vi "Agilent VNA Read Measurement.vi"(6 "Channel":i8=1 min=1 max=99 step=1, 7 "Agilent VNA":T2, 8 "error in (no error)":errorcluster, 11 "VISA Resource Name":refnum<visa-resource-name>) -> (0 "error out":errorcluster, 1 "Parameter":T1 {"Stimulus Port" min=1 step=1; "Response Port" min=1 step=1}, 2 "Measurement":T3=enum."Analog In - Aux In", 3 "dup VISA Resource Name":refnum<visa-resource-name>)   [LabVIEW 2011]
doc: "This VI for the HP 8753B is used to read the meausurement format.\n\n0 log magnitude\n1 phase\n2 delay\n3 Smith chart\n4 polar\n5 linear magnitude\n6 standing wave ratio\n7 real\n8 imaginary"
uses:
  TypeDefs/Agilent VNA Measurement.ctl
  TypeDefs/Agilent VNA Instrument Info.ctl
  tests/S Parameter/TypeDefs/SP Parameter.ctl
panel:
  in  "Trace":i8=1 min=1 max=99 step=1
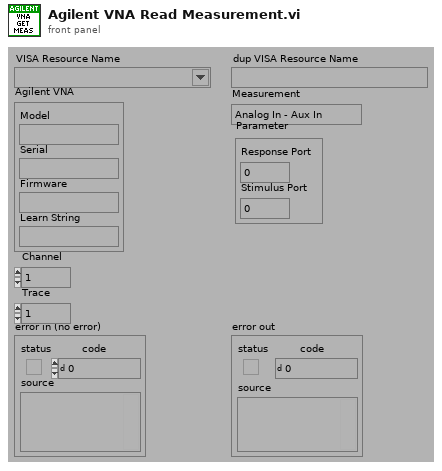
[diagram p1: front panel]
types:
  T1 = typedef "SP Parameter.ctl" = cluster{"Stimulus Port":i8, "Response Port":i8}
  T2 = typedef "Agilent VNA Instrument Info.ctl" = cluster{"Model":string, "Serial":string, "Firmware":string, "Learn String":string}
  T3 = typedef "Agilent VNA Measurement.ctl" = enum32{"SXX", "Analog In - Aux In", "A/R", "B/R", "A/B", "A", "B", "R"}
  T4 = typedef "Agilent VNA Model.ctl" = enum16{"Not Supported", "8510X", "8719X", "8720X", "8722X", "8753X", "ENA", "PNA", "Field Fox"}
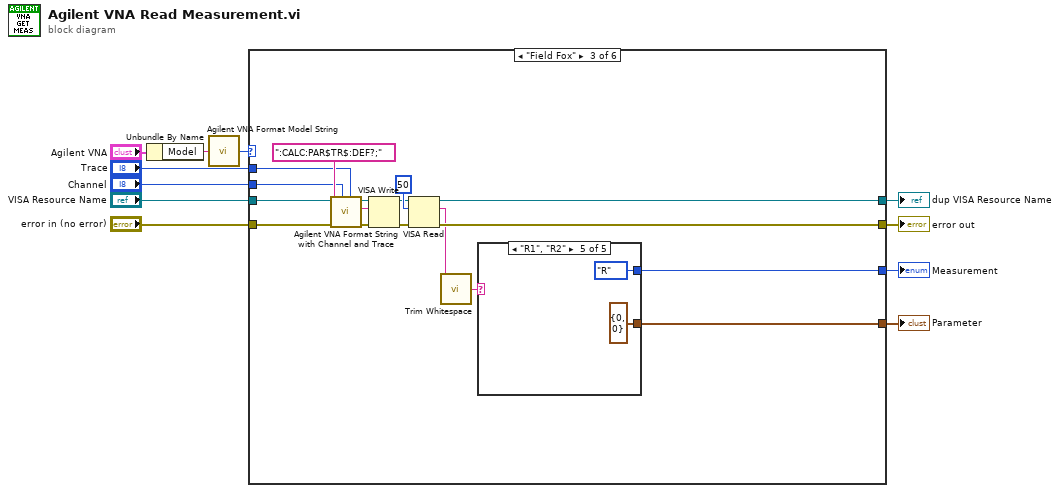
[diagram p0: block diagram]
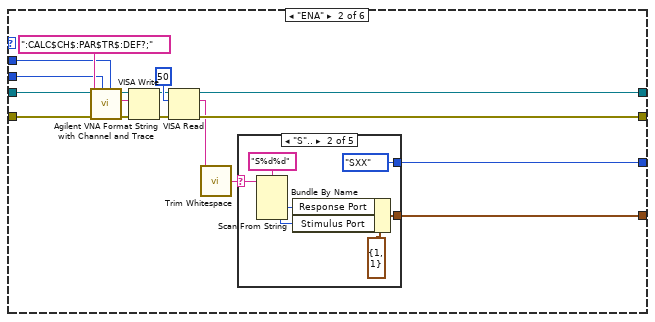
[diagram p3: hidden frame]
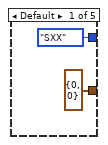
[diagram p4: hidden frame]
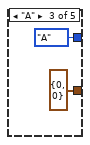
[diagram p5: hidden frame]
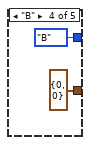
[diagram p6: hidden frame]
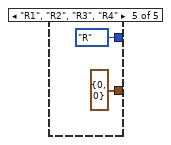
[diagram p7: hidden frame]
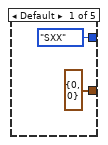
[diagram p8: hidden frame]
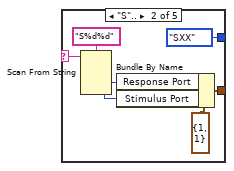
[diagram p9: hidden frame]
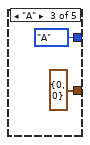
[diagram p10: hidden frame]
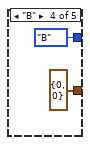
[diagram p11: hidden frame]
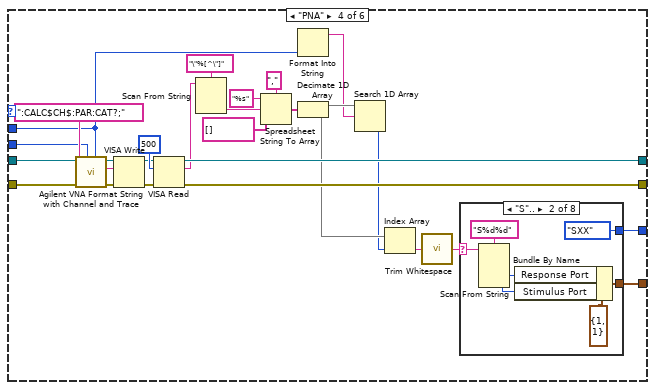
[diagram p12: hidden frame]
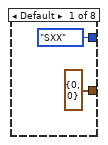
[diagram p13: hidden frame]
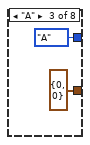
[diagram p14: hidden frame]
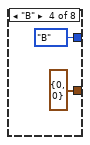
[diagram p15: hidden frame]
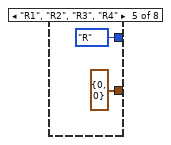
[diagram p16: hidden frame]
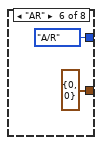
[diagram p17: hidden frame]
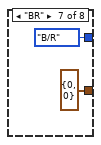
[diagram p18: hidden frame]
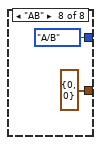
[diagram p19: hidden frame]
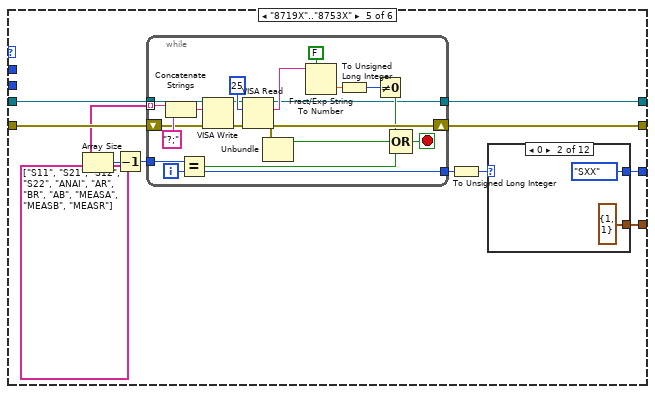
[diagram p20: hidden frame]
diagram:
  n1 = Unbundle By Name("Agilent VNA") -> ("Model"=w2:string)
  n2 = call "Agilent VNA Format Model String.vi"("Model"=w2) -> ("Model"=w6:T4)
  n3 = case shown="\"Field Fox\"" w6 {
    tunnel: "VISA Resource Name" -> [w12 w22 w52 w93 w131 w188]
    tunnel: "error in (no error)" -> [w13 w26 w56 w97 w130 w187]
    tunnel: [w13 w24 w54 w95 w127 w186] -> w9
    tunnel: [_ w17 w47 w75 w122 w177] -> w8
    tunnel: [w12 w23 w53 w94 w124 w185] -> w7
    tunnel: "Channel" -> [_ w16 w46 w78 _ _]
    tunnel: "Trace" -> [_ w15 w45 w77 _ _]
    tunnel: [_ w14 w44 w76 w123 w178] -> w1
    frame "Not Supported" {
    }
    frame "ENA" {
      n4 = call "Agilent VNA Format String with Channel and Trace.vi"("Trace"=w15, "Channel"=w16, "String"=":CALC$CH$:PAR$TR$:DEF?;") -> ("String Out"=w20:string)  [unwired: 6 out]
      n5 = VISA Write(VISA resource name=w22, write buffer=w20, error in (no error)=w26) -> (VISA resource name out=w27:refnum<visa-resource-name>, error out=w25:errorcluster)  [unwired: 1 out]
      n6 = VISA Read(VISA resource name=w27, byte count=u32 50, error in (no error)=w25) -> (VISA resource name out=w23:refnum<visa-resource-name>, read buffer=w19:string, error out=w24:errorcluster)  [unwired: 1 out]
      n7 = call <vilib>:"Trim Whitespace.vi"("string"=w19) -> ("trimmed string"=w18:string)  [unwired: 1 in]
      n8 = case shown="\"S\".." w18 {
        selector: w18 -> [_ w36 _ _ _]
        tunnel: [Agilent_VNA_Measurement."SXX" ("Display Format") Agilent_VNA_Measurement."SXX" ("Display Format") Agilent_VNA_Measurement."A" ("Display Format") Agilent_VNA_Measurement."B" ("Display Format") Agilent_VNA_Measurement."R" ("Display Format")] -> w17
        tunnel: [T1 {"Stimulus Port"=0, "Response Port"=0} ("Parameter") w33 T1 {"Stimulus Port"=0, "Response Port"=0} ("Parameter") T1 {"Stimulus Port"=0, "Response Port"=0} ("Parameter") T1 {"Stimulus Port"=0, "Response Port"=0} ("Parameter")] -> w14
        frame Default {
        }
        frame "S".. {
          n9 = Scan From String(format string="S%d%d", input string=w36) -> (output 1=w32:i32, output 2=w31:i32)  [unwired: 2 in, 5 out]
          n10 = Bundle By Name(cluster=T1 {"Stimulus Port"=1, "Response Port"=1} ("Parameter"), "Response Port"=w32, "Stimulus Port"=w31) -> (w33:T1)
        }
        frame "A" {
        }
        frame "B" {
        }
        frame "R1", "R2", "R3", "R4" {
        }
      }
    }
    frame "Field Fox" {
      n11 = call "Agilent VNA Format String with Channel and Trace.vi"("Trace"=w45, "Channel"=w46, "String"=":CALC:PAR$TR$:DEF?;") -> ("String Out"=w50:string)  [unwired: 6 out]
      n12 = VISA Write(VISA resource name=w52, write buffer=w50, error in (no error)=w56) -> (VISA resource name out=w57:refnum<visa-resource-name>, error out=w55:errorcluster)  [unwired: 1 out]
      n13 = VISA Read(VISA resource name=w57, byte count=u32 50, error in (no error)=w55) -> (VISA resource name out=w53:refnum<visa-resource-name>, read buffer=w49:string, error out=w54:errorcluster)  [unwired: 1 out]
      n14 = call <vilib>:"Trim Whitespace.vi"("string"=w49) -> ("trimmed string"=w48:string)  [unwired: 1 in]
      n15 = case shown="\"R1\", \"R2\"" w48 {
        selector: w48 -> [_ w66 _ _ _]
        tunnel: [Agilent_VNA_Measurement."SXX" ("Display Format") Agilent_VNA_Measurement."SXX" ("Display Format") Agilent_VNA_Measurement."A" ("Display Format") Agilent_VNA_Measurement."B" ("Display Format") Agilent_VNA_Measurement."R" ("Display Format")] -> w47
        tunnel: [T1 {"Stimulus Port"=0, "Response Port"=0} ("Parameter") w63 T1 {"Stimulus Port"=0, "Response Port"=0} ("Parameter") T1 {"Stimulus Port"=0, "Response Port"=0} ("Parameter") T1 {"Stimulus Port"=0, "Response Port"=0} ("Parameter")] -> w44
        frame Default {
        }
        frame "S".. {
          n16 = Scan From String(format string="S%d%d", input string=w66) -> (output 1=w62:i32, output 2=w61:i32)  [unwired: 2 in, 5 out]
          n17 = Bundle By Name(cluster=T1 {"Stimulus Port"=1, "Response Port"=1} ("Parameter"), "Response Port"=w62, "Stimulus Port"=w61) -> (w63:T1)
        }
        frame "A" {
        }
        frame "B" {
        }
        frame "R1", "R2" {
        }
      }
    }
    frame "PNA" {
      n18 = call "Agilent VNA Format String with Channel and Trace.vi"("Trace"=w77, "Channel"=w78, "String"=":CALC$CH$:PAR:CAT?;") -> ("String Out"=w91:string)  [unwired: 6 out]
      n19 = VISA Write(VISA resource name=w93, write buffer=w91, error in (no error)=w97) -> (VISA resource name out=w98:refnum<visa-resource-name>, error out=w96:errorcluster)  [unwired: 1 out]
      n20 = VISA Read(VISA resource name=w98, byte count=u32 500, error in (no error)=w96) -> (VISA resource name out=w94:refnum<visa-resource-name>, read buffer=w85:string, error out=w95:errorcluster)  [unwired: 1 out]
      n21 = Scan From String(format string="\"%[^\"]", input string=w85) -> (output 1=w87:string)  [unwired: 2 in, 4 out]
      n22 = Spreadsheet String To Array(delimiter (Tab)=",", format string="%s", spreadsheet string=w87, array type (2D Dbl)=string[] []) -> (array=w84:string[])
      n23 = Format Into String(w77) -> (resulting string=w82:string)  [unwired: 3 in, 1 out]
      n24 = Decimate 1D Array(w84) -> (w83:string[], w81:string[])
      n25 = Search 1D Array(1D array=w83, element=w82) -> (index of element=w80:i32)  [unwired: 1 out]
      n26 = Index Array(array=w81, index=w80) -> (element=w79:string)
      n27 = call <vilib>:"Trim Whitespace.vi"("string"=w79) -> ("trimmed string"=w74:string)  [unwired: 1 in]
      n28 = case shown="\"S\".." w74 {
        selector: w74 -> [_ w107 _ _ _ _ _ _]
        tunnel: [Agilent_VNA_Measurement."SXX" ("Display Format") Agilent_VNA_Measurement."SXX" ("Display Format") Agilent_VNA_Measurement."A" ("Display Format") Agilent_VNA_Measurement."B" ("Display Format") Agilent_VNA_Measurement."R" ("Display Format") Agilent_VNA_Measurement."A/R" ("Display Format") Agilent_VNA_Measurement."B/R" ("Display Format") Agilent_VNA_Measurement."A/B" ("Display Format")] -> w75
        tunnel: [T1 {"Stimulus Port"=0, "Response Port"=0} ("Parameter") w104 T1 {"Stimulus Port"=0, "Response Port"=0} ("Parameter") T1 {"Stimulus Port"=0, "Response Port"=0} ("Parameter") T1 {"Stimulus Port"=0, "Response Port"=0} ("Parameter") T1 {"Stimulus Port"=0, "Response Port"=0} ("Parameter") T1 {"Stimulus Port"=0, "Response Port"=0} ("Parameter") T1 {"Stimulus Port"=0, "Response Port"=0} ("Parameter")] -> w76
        frame Default {
        }
        frame "S".. {
          n29 = Scan From String(format string="S%d%d", input string=w107) -> (output 1=w103:i32, output 2=w102:i32)  [unwired: 2 in, 5 out]
          n30 = Bundle By Name(cluster=T1 {"Stimulus Port"=1, "Response Port"=1} ("Parameter"), "Response Port"=w103, "Stimulus Port"=w102) -> (w104:T1)
        }
        frame "A" {
        }
        frame "B" {
        }
        frame "R1", "R2", "R3", "R4" {
        }
        frame "AR" {
        }
        frame "BR" {
        }
        frame "AB" {
        }
      }
    }
    frame "8719X".."8753X" {
      w129 = string[] ["S11", "S21", "S12", "S22", "ANAI", "AR", "BR", "AB", "MEASA", "MEASB", "MEASR"]
      n31 = Array Size(array=w129) -> (size(s)=w128:i32)
      n32 = Decrement(x=w128) -> (x-1=w126:i32)
      n33 = while {
        tunnel: w131 -> [w172]
        shift-right: [w163] -> w127
        shift-left: w130 -> [w164]
        tunnel: w129 -> [w165] mode=indexing
        tunnel: w126 -> [w162]
        tunnel: [w157] -> w125
        tunnel: [w156] -> w124
        i -> [w157]
        stop <- w158 stop-if-true
        n34 = Concatenate Strings(w165, "?;") -> (w166:string)
        n35 = Equal?(x=w162, y=w157) -> (x = y?=w161:bool)
        n36 = VISA Write(VISA resource name=w172, write buffer=w166, error in (no error)=w164) -> (VISA resource name out=w173:refnum<visa-resource-name>, error out=w175:errorcluster)  [unwired: 1 out]
        n37 = VISA Read(VISA resource name=w173, byte count=u32 25, error in (no error)=w175) -> (VISA resource name out=w156:refnum<visa-resource-name>, read buffer=w170:string, error out=w163:errorcluster)  [unwired: 1 out]
        n38 = Unbundle(w163) -> ("status"=w160:bool)  [unwired: 2 out]
        n39 = Fract/Exp String To Number(use system decimal point (T)=FALSE, string=w170) -> (number=w171:dbl)  [unwired: 3 out]
        n40 = To Unsigned Long Integer(number=w171) -> (unsigned 32bit integer=w168:u32)
        n41 = Not Equal To 0?(x=w168) -> (x != 0?=w159:bool)
        n42 = Compound Arithmetic op=OR(w159, w160, w161) -> (w158:bool)
      }
      n43 = To Unsigned Long Integer(number=w125) -> (unsigned 32bit integer=w121:u32)
      n44 = case shown="0" w121 {
        tunnel: [Agilent_VNA_Measurement."SXX" ("Display Format") Agilent_VNA_Measurement."SXX" ("Display Format") Agilent_VNA_Measurement."SXX" ("Display Format") Agilent_VNA_Measurement."SXX" ("Display Format") Agilent_VNA_Measurement."SXX" ("Display Format") Agilent_VNA_Measurement."Analog In - Aux In" ("Display Format") Agilent_VNA_Measurement."A/R" ("Display Format") Agilent_VNA_Measurement."B/R" ("Display Format") Agilent_VNA_Measurement."A/B" ("Display Format") Agilent_VNA_Measurement."A" ("Display Format") Agilent_VNA_Measurement."B" ("Display Format") Agilent_VNA_Measurement."R" ("Display Format")] -> w122
        tunnel: [T1 {"Stimulus Port"=0, "Response Port"=0} ("Parameter") T1 {"Stimulus Port"=1, "Response Port"=1} ("Parameter") T1 {"Stimulus Port"=1, "Response Port"=2} ("Parameter") T1 {"Stimulus Port"=2, "Response Port"=1} ("Parameter") T1 {"Stimulus Port"=2, "Response Port"=2} ("Parameter") T1 {"Stimulus Port"=0, "Response Port"=0} ("Parameter") T1 {"Stimulus Port"=0, "Response Port"=0} ("Parameter") T1 {"Stimulus Port"=0, "Response Port"=0} ("Parameter") T1 {"Stimulus Port"=0, "Response Port"=0} ("Parameter") T1 {"Stimulus Port"=0, "Response Port"=0} ("Parameter") T1 {"Stimulus Port"=0, "Response Port"=0} ("Parameter") T1 {"Stimulus Port"=0, "Response Port"=0} ("Parameter")] -> w123
        frame Default {
        }
        frame 0 {
        }
        frame 1 {
        }
        frame 2 {
        }
        frame 3 {
        }
        frame 4 {
        }
        frame 5 {
        }
        frame 6 {
        }
        frame 7 {
        }
        frame 8 {
        }
        frame 9 {
        }
        frame 10 {
        }
      }
    }
    frame "8510X" {
      n45 = VISA Write(VISA resource name=w188, write buffer="PARA?;", error in (no error)=w187) -> (VISA resource name out=w182:refnum<visa-resource-name>, error out=w184:errorcluster)  [unwired: 1 out]
      n46 = VISA Read(VISA resource name=w182, byte count=u32 25, error in (no error)=w184) -> (VISA resource name out=w185:refnum<visa-resource-name>, read buffer=w180:string, error out=w186:errorcluster)  [unwired: 1 out]
      n47 = call <vilib>:"Trim Whitespace.vi"("string"=w180) -> ("trimmed string"=w179:string)  [unwired: 1 in]
      n48 = call "Strip Quotes From String.vi"("String In"=w179) -> ("Trimmed String"=w176:string)
      n49 = case shown="\"S\".." w176 {
        selector: w176 -> [_ w197]
        tunnel: [Agilent_VNA_Measurement."SXX" ("Display Format") Agilent_VNA_Measurement."SXX" ("Display Format")] -> w177
        tunnel: [T1 {"Stimulus Port"=0, "Response Port"=0} ("Parameter") w194] -> w178
        frame Default {
        }
        frame "S".. {
          n50 = Scan From String(format string="S%d%d", input string=w197) -> (output 1=w193:i32, output 2=w192:i32)  [unwired: 2 in, 5 out]
          n51 = Bundle By Name(cluster=T1 {"Stimulus Port"=1, "Response Port"=1} ("Parameter"), "Response Port"=w193, "Stimulus Port"=w192) -> (w194:T1)
        }
      }
    }
  }
  "Measurement" <- w8
  "dup VISA Resource Name" <- w7
  "error out" <- w9
  "Parameter" <- w1
